vi "Linear JTFA Method.vi"() -> ()   [LabVIEW 2019]
doc: "This example shows the signal processing procedure of linear time-frequency analysis methods. In practice, the procedure includes the following steps:\n\n1) Perform a linear transform on a signal, such as the STFT, the Gabor transform, and the adaptive transform.\n2) Process the result of the transform by filtering, thresholding, masking, or by other analysis methods.\n3) Reconstruct the signal with the inverse STFT, the Gabor expansion, or the adaptive expansion.\n\nThis example computes the linear time-frequency representation of a signal by using the TFA Discrete Gabor Transform VI; processes the linear time-frequency representation by using the thresholding method; and reconstructs the time domain signal from the processed linear time-frequency representation by using the TFA Discrete Gabor Expansion VI.\n\n<b>Instructions:</b>\n1) Run this VI continuously.\n2) Move the <b>Thresholding Factor</b> slide control.\n3) Observe the <b>Reconstructed Signal</b> in the flowchart."
uses:
  <vilib>/addons/Time Frequency Analysis/typedefs.llb/TFA Data.ctl
  Instance           7 26Saved   Linear JTFA Method .vi
  <vilib>/addons/Time Frequency Analysis/Transform.llb/TFA Discrete Gabor Transform (Waveform).vi
  <vilib>/addons/Time Frequency Analysis/Transform.llb/TFA Discrete Gabor Expansion (Waveform).vi
  <vilib>/addons/_Advanced Signal Processing/NI_AdvSigProcTFA.lvlib
panel:
  out "aspt-left-top":bool
  out "Gabor Coefficients":dbl[][](graph)
  in  "Thresholding Factor":dbl(slide)=0.494949494949495 scale=0.0..1.0
  out "Reconstructed Signal":waveform(dbl)(graph)
  out "Processed Gabor Coefficients":dbl[][](graph)
  out "Source Signal":waveform(dbl)(graph)
  # "Overview: Shows the signal processing procedure of linear time-frequency analysis methods. \nRequirements: LabVIEW Full Development System, Advanced Signal Processing Toolkit\nInstructions: \n1. Run this VI continuously.\n2. Move the Thresholding Factor slide control.\n3. Observe the Reconstructed Signal in the flowchart."
  # "Transform"
  # "Reconstruction"
  # "Processing (E.g., thresholding)"
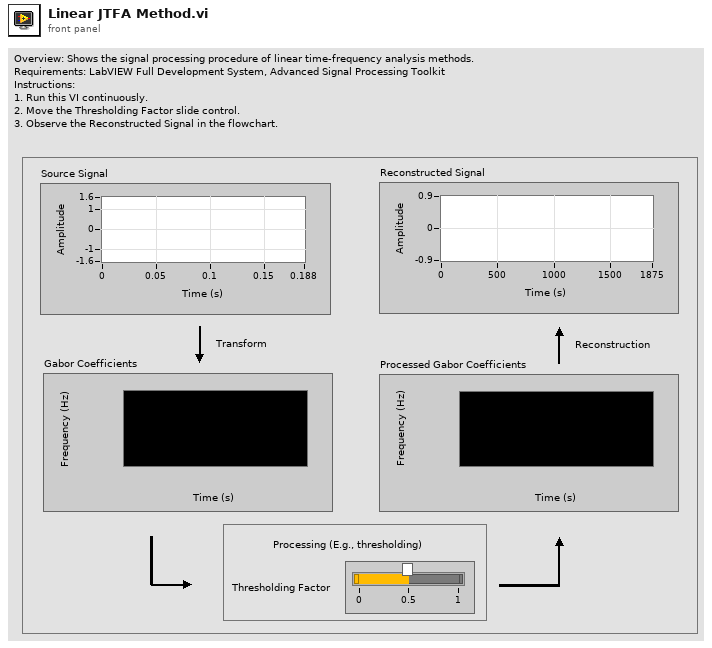
[diagram p1: front panel]
types:
  T1 = typedef "NI_AdvSigProcTFA.lvlib/TFA Data.ctl" = u16
  T2 = cluster{"synthesis window":dbl[], "dM (time steps)":i32, "N (frequency bins)":i32}
  T3 = cluster{"analysis window":dbl[], "dM (time steps)":i32, "N (frequency bins)":i32}
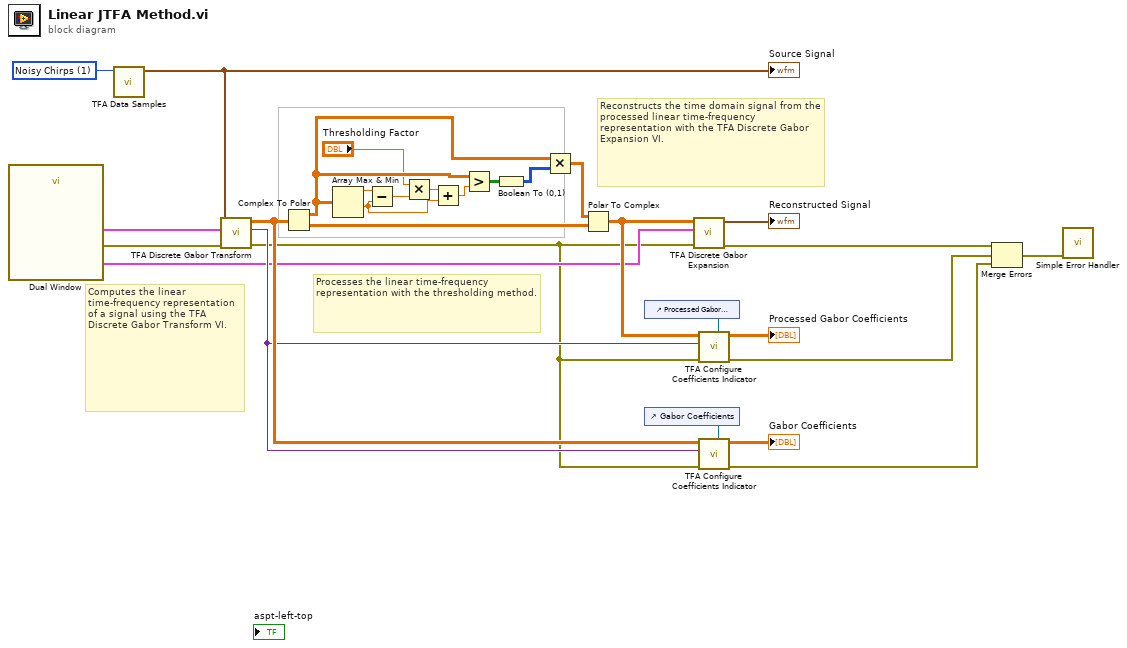
[diagram p0: block diagram]
diagram:
  w7 = T1 1 items=["PC Fan"=0, "Noisy Chirps"=1, "TDR 1"=2, "TDR 2"=3, "Liquefaction"=4, "Liquefaction Free"=5, "Aneurysm"=6, "Bat"=7, "RF"=8, "Two Gaussian"=9, "Three Gaussian"=10, "Chirp"=11, "Gaussian Chirp"=12, "Cross Chirp"=13, "Doppler"=14, "HOP"=15, "TF Sine"=16, "Three Tone"=17, "Four Tone"=23, "Blood Flow Doppler (phase a)"=20, "Blood Flow Doppler (phase b)"=21, "Heart sound"=22, "-"=18, "Random Noise"=19] ("data")
  # "Reconstructs the time domain signal from the processed linear time-frequency representation with the TFA Discrete Gabor Expansion VI."
  # "Processes the linear time-frequency representation with the thresholding method."
  # "Computes the linear time-frequency representation of a signal using the TFA Discrete Gabor Transform VI."
  n1 = call "Dual Window"() -> ("error out"=w1:errorcluster, "expansion info"=w8:T2, "transform info"=w9:T3)  [unwired: 1 in, 8 out]
  n2 = call <vilib>:"TFA Data Samples.vi"("data"=w7) -> ("signal"=w28:waveform(dbl))  [unwired: 10 out]
  "Source Signal" <- w28
  n3 = call-poly <vilib>:"TFA Discrete Gabor Transform.vi"("error in (no error)"=w1, "transform info"=w9, "signal"=w28) -> ("error out"=w6:errorcluster, "scale info"=w12:variant, "Gabor coef"=w13:cdb[][])  [unwired: 6 out]
  n4 = Complex To Polar(r * e^(i*theta)=w13) -> (r=w18:dbl[][], theta=w27:dbl[][])
  n5 = Array Max & Min(array=w18) -> (max value=w26:dbl, min value=w23:dbl)  [unwired: 2 out]
  n6 = Subtract(x=w26, y=w23) -> (x-y=w25:dbl)
  n7 = Multiply(x="Thresholding Factor", y=w25) -> (x*y=w24:dbl)
  n8 = Add(x=w24, y=w23) -> (x+y=w19:dbl)
  n9 = Greater?(x=w18, y=w19) -> (0:w22:bool[][])
  n10 = Boolean To (0,1)(Boolean=w22) -> (0, 1=w20:i16[][])
  n11 = Multiply(x=w18, y=w20) -> (x*y=w21:dbl[][])
  n12 = Polar To Complex(1:w27, 2:w21) -> (0:w16:cdb[][])
  n13 = control-ref of="Processed Gabor Coefficients"() -> (w14:refnum<vi>)
  n14 = control-ref of="Gabor Coefficients"() -> (w10:refnum<vi>)
  n15 = call-poly <vilib>:"TFA Discrete Gabor Expansion.vi"("error in (no error)"=w6, "expansion info"=w8, "Gabor coef"=w16) -> ("error out"=w5:errorcluster, "signal"=→"Reconstructed Signal":waveform(dbl))  [unwired: 7 out]
  n16 = call <vilib>:"TFA Configure Coefficients Indicator.vi"("reference of TF coefficients indicator"=w14, "error in (no error)"=w6, "scale info"=w12, "TF coefficients"=w16) -> ("error out"=w4:errorcluster, "TF coefficients indicator"=→"Processed Gabor Coefficients":dbl[][])  [unwired: 3 in, 3 out]
  n17 = call <vilib>:"TFA Configure Coefficients Indicator.vi"("reference of TF coefficients indicator"=w10, "error in (no error)"=w6, "scale info"=w12, "TF coefficients"=w13) -> ("error out"=w3:errorcluster, "TF coefficients indicator"=→"Gabor Coefficients":dbl[][])  [unwired: 3 in, 3 out]
  n18 = Merge Errors(w5, w4, w3) -> (w2:errorcluster)
  n19 = call <vilib>:"Simple Error Handler.vi"("error in (no error)"=w2) -> ()  [unwired: 4 in, 5 out]
